vi "SetSourceLevel.vi"(7 "SMU":T2, 8 "Error In":errorcluster, 9 "Level (V or A)":dbl=1.0, 10 "Source Function":T1, 11 "Keithley 2602 In":refnum<visa-resource-name>) -> (0 "Error Out":errorcluster, 3 "Keithley 2602 Out":refnum<visa-resource-name>)   [LabVIEW 2013, in "Keithley-2602.lvlib"]
uses:
  Keithley-2602.lvlib
  Controls/SMU.ctl
  Controls/SourceFunction.ctl
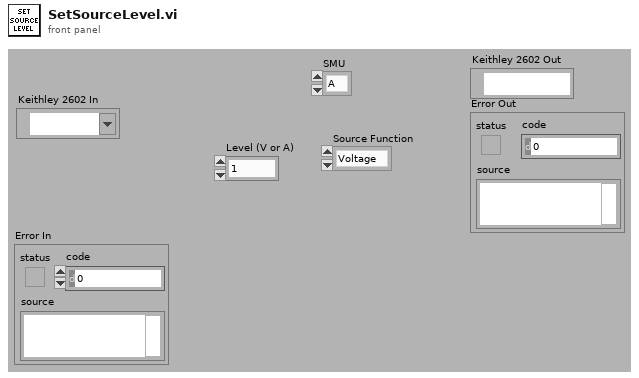
[diagram p1: front panel]
types:
  T1 = typedef "Keithley-2602.lvlib/SourceFunction.ctl" = enum16{"Voltage", "Current"}
  T2 = typedef "Keithley-2602.lvlib/SMU.ctl" = enum16{"A", "B"}
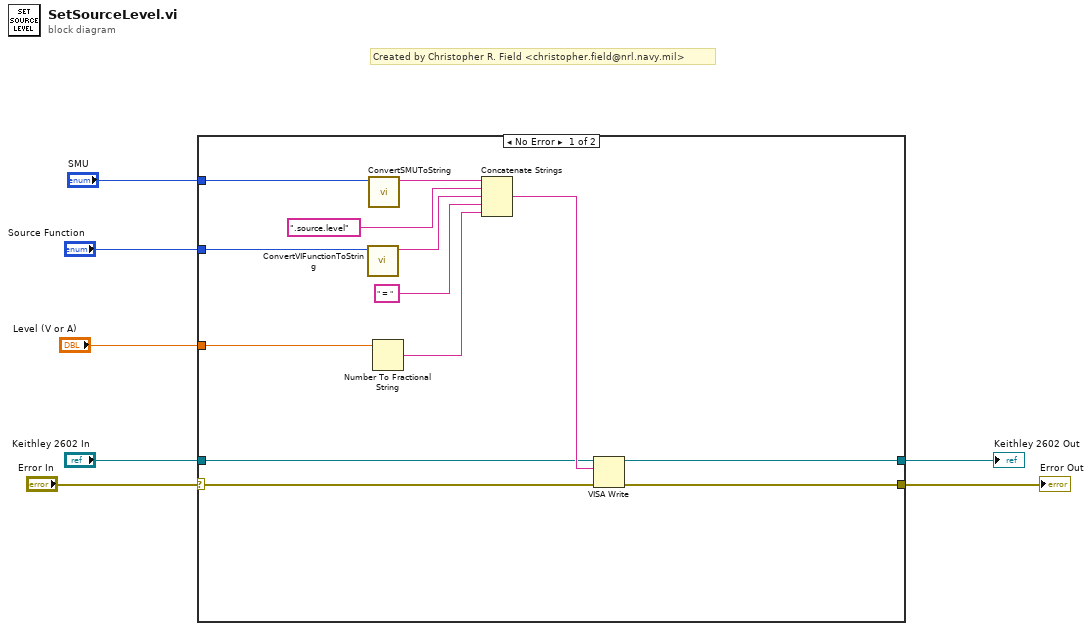
[diagram p0: block diagram]
diagram:
  # "Created by Christopher R. Field <christopher.field@nrl.navy.mil>"
  n1 = case shown="No Error" "Error In" {
    selector: "Error In" -> [w8 w21]
    tunnel: "Keithley 2602 In" -> [w18 w22]
    tunnel: [w17 w22] -> w6
    tunnel: [w16 w21] -> w5
    tunnel: "Level (V or A)" -> [w12 _]
    tunnel: "SMU" -> [w10 _]
    tunnel: "Source Function" -> [w9 _]
    frame No Error {
      n2 = call "ConvertVIFunctionToString.vi"("Function"=w9) -> ("Function (v or i)"=w13:string)  [unwired: 10 in]
      n3 = call "ConvertSMUToString.vi"("SMU"=w10) -> ("Channel"=w14:string)  [unwired: 10 in]
      n4 = Number To Fractional String(number=w12) -> (F-format string=w11:string)  [unwired: 3 in]
      n5 = Concatenate Strings(w14, ".source.level", w13, " = ", w11) -> (w19:string)
      n6 = VISA Write(VISA resource name=w18, write buffer=w19, error in (no error)=w8) -> (VISA resource name out=w17:refnum<visa-resource-name>, error out=w16:errorcluster)  [unwired: 1 out]
    }
    frame Error {
    }
  }
  "Keithley 2602 Out" <- w6
  "Error Out" <- w5
